vi "SetTensionerPosition.vi"(10 "LoopCount":i32) -> ()   [LabVIEW 2015]
uses:
  Utilities/MotorPositionGlobals.vi
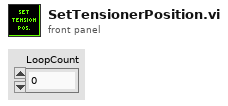
[diagram p1: front panel]
types:
  T1 = typedef "WPI_MotorControlDeviceRef.ctl" = cluster{"DeviceStatus":errorcluster, "Type":T2, "PWM":cluster{"PWM Channel":T3, "DeadBand":T4}, "CAN":cluster{"Device Number":u8, "Control Mode":T5, "Semaphore":T6, "Max Vout":dbl, "TalonSRX Control Mode":T7}, "Invert":bool}
  T2 = typedef "WPI_MotorControlType.ctl" = enum16{"PWM", "CAN", "CANTalonSRX"}
  T3 = typedef "FPGA_DIOPWMChannel.ctl" = enum8{"PWM 0", "PWM 1", "PWM 2", "PWM 3", "PWM 4", "PWM 5", "PWM 6", "PWM 7", "PWM 8", "PWM 9", "PWM MXP 0", "PWM MXP 1", "PWM MXP 2", "PWM MXP 3", "PWM MXP 4", "PWM MXP 5", "PWM MXP 6", "PWM MXP 7", "PWM MXP 8", "PWM MXP 9", "Invalid"}
  T4 = typedef "WPI_PWMDeadband.ctl" = cluster{"Name":string, "maxPositivePwm":i32, "minPositivePwm":i32, "centerPwm":i32, "maxNegativePwm":i32, "minNegativePwm":i32, "angularRange":u16}
  T5 = typedef "WPI_CANJaguar_ControlMode.ctl" = enum8{"Percent VBus", "Current", "Speed", "Position", "Voltage"}
  T6 = typedef "Semaphore RefNum" = refnum<k1>
  T7 = typedef "WPI_CANTalonSRX_APIControlMode.ctl" = enum8{"Percent VBus", "Speed", "Position", "Slave", "Unchanged / Invalid", "Voltage Compensation", "Current", "Motion Profile"}
  T8 = typedef "WPI_SwitchDevRef.ctl" = cluster{"DevStatus":errorcluster, "DIO Channel":T9, "CntIndex":T10, "Normally Closed":bool}
  T9 = typedef "FPGA_DIOChannel.ctl" = enum8{"DIO 0", "DIO 1", "DIO 2", "DIO 3", "DIO 4", "DIO 5", "DIO 6", "DIO 7", "DIO 8", "DIO 9", "DIO MXP 0", "DIO MXP 1", "DIO MXP 2", "DIO MXP 3", "DIO MXP 4", "DIO MXP 5", "DIO MXP 6", "DIO MXP 7", "DIO MXP 8", "DIO MXP 9", "DIO MXP 10", "DIO MXP 11", "DIO MXP 12", "DIO MXP 13", "DIO MXP 14", "DIO MXP 15", "Invalid"}
  T10 = typedef "FPGA_CounterCtrSystemIndex.ctl" = enum8{"Ctr 0", "Ctr 1", "Ctr 2", "Ctr 3", "Ctr 4", "Ctr 5", "Ctr 6", "Ctr 7", "Invalid"}
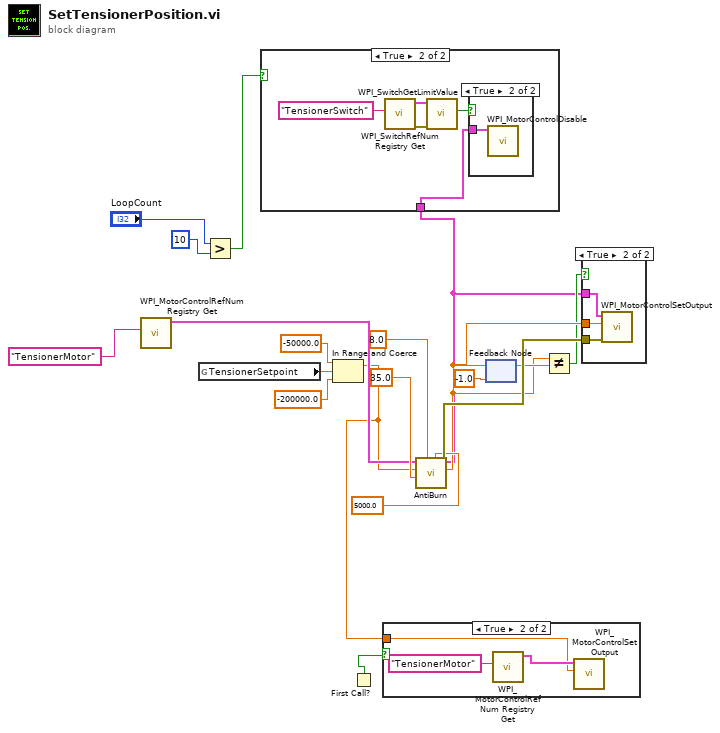
[diagram p0: block diagram]
diagram:
  n1 = call <vilib>:"WPI_MotorControlRefNum Registry Get.vi"("refnum name"="TensionerMotor") -> ("MotorControlDevRef"=w3:T1)  [unwired: 9 in, 1 out]
  n2 = global read "MotorPositionGlobals.vi" "TensionerSetpoint"() -> (w19:dbl)
  n3 = Greater?(x="LoopCount", y=10 ("LoopCount")) -> (0:w7:bool)
  n4 = In Range and Coerce(upper limit=-50000.0, x=w19, lower limit=-200000.0) -> (coerced(x)=w1:dbl)  [unwired: 1 out]
  n5 = First Call?() -> (First Call?: T/F=w2:bool)
  n6 = case shown="True" w2 {
    tunnel: w1 -> [_ w20]
    frame False {
    }
    frame True {
      n7 = call <vilib>:"WPI_MotorControlRefNum Registry Get.vi"("refnum name"="TensionerMotor") -> ("MotorControlDevRef"=w21:T1)  [unwired: 9 in, 1 out]
      n8 = call <vilib>:"WPI_MotorControlSetOutput.vi"("Output"=w20, "MotorControlDevRef"=w21) -> ()  [unwired: 7 in, 3 out]
    }
  }
  n9 = call "AntiBurn.vi"("AllowedEncoderError"=5000.0, "AllowedTimeDeviation"=8.0, "MaxCurrent"=35.0, "MotorSetpoint"=w1, "CAN Talon SRX Ref"=w3) -> ("error out"=w16:errorcluster, "MotorSetpointOut"=w11:dbl, "MotorControlDevRef"=w8:T1)  [unwired: 3 in, 1 out]
  n10 = case shown="True" w7 {
    tunnel: w8 -> [_ w23]
    frame False {
    }
    frame True {
      n11 = call <vilib>:"WPI_SwitchRefNum Registry Get.vi"("refnum name"="TensionerSwitch") -> ("error out"=w25:errorcluster, "SwitchDevRef"=w26:T8)  [unwired: 9 in]
      n12 = call <vilib>:"WPI_SwitchGetLimitValue.vi"("error in (no error)"=w25, "SwitchDevRef"=w26) -> ("Switch Pressed"=w24:bool)  [unwired: 7 in, 2 out]
      n13 = case shown="True" w24 {
        tunnel: w23 -> [_ w28]
        frame False {
        }
        frame True {
          n14 = call <vilib>:"WPI_MotorControlDisable.vi"("MotorControlDevRef"=w28) -> ()  [unwired: 9 in, 2 out]
        }
      }
    }
  }
  n15 = feedback-in #1(w11) -> ()
  n16 = feedback #1(-1.0 ("MotorSetpointOut")) -> (w12:dbl)
  n17 = Not Equal?(x=w11, y=w12) -> (x != y?=w10:bool)
  n18 = case shown="True" w10 {
    tunnel: w8 -> [_ w31]
    tunnel: w11 -> [_ w30]
    tunnel: w16 -> [_ w29]
    frame False {
    }
    frame True {
      n19 = call <vilib>:"WPI_MotorControlSetOutput.vi"("error in (no error)"=w29, "Output"=w30, "MotorControlDevRef"=w31) -> ()  [unwired: 6 in, 3 out]
    }
  }
